vi "scale.vi"(10 "dt":dbl=1e-07, 11 "waveforms":dbl[][](array[numeric])=array5x1000[5000 elements]) -> (2 "el":waveform(dbl)[](graph))   [LabVIEW 2017, in "wf.lvlib" / "wf_tools.lvlib"]
uses:
  wf_tools.lvlib
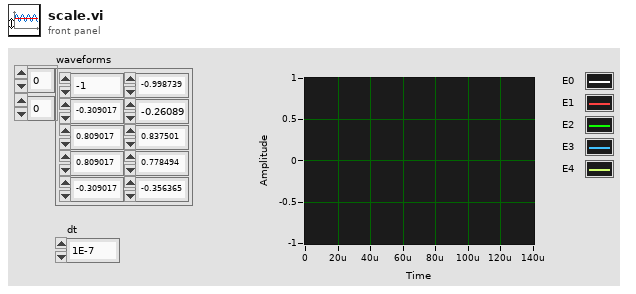
[diagram p1: front panel]
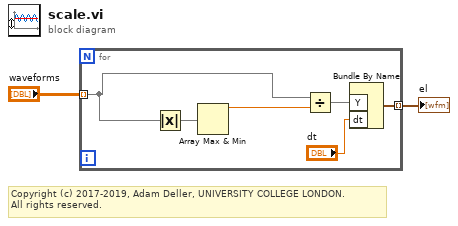
[diagram p0: block diagram]
diagram:
  # "Copyright (c) 2017-2019, Adam Deller, UNIVERSITY COLLEGE LONDON.\nAll rights reserved."
  n1 = for {
    tunnel: "waveforms" -> [w5] mode=indexing
    tunnel: [w7] -> w1 mode=indexing
    n2 = Absolute Value(x=w5) -> (abs(x)=w4:dbl[])
    n3 = Array Max & Min(array=w4) -> (max value=w3:dbl)  [unwired: 3 out]
    n4 = Divide(x=w5, y=w3) -> (x/y=w6:dbl[])
    n5 = Bundle By Name("Y"=w6, "dt"="dt") -> (w7:waveform(dbl))  [unwired: 1 in]
  }
  "el" <- w1
